vi "Heat1D_Cal Coeff.vi"(9 "a":dbl, 10 "k":dbl=1.0, 11 "Domain":T1) -> (2 "Coefficients":cluster{"r":dbl, "s":dbl, "dt":dbl, "dx":dbl}, 3 "Domain Dup":T1)   [LabVIEW 2017, in "NI_PDE.lvlib"]
uses:
  <vilib>/gmath/NI_PDE.lvlib
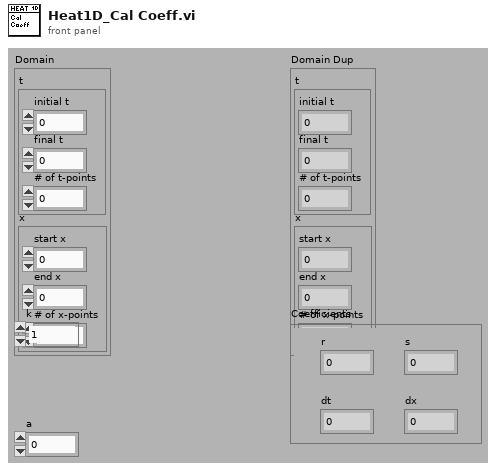
[diagram p1: front panel]
types:
  T1 = cluster{"t":cluster{"initial t":dbl, "final t":dbl, "# of t-points":i32}, "x":cluster{"start x":dbl, "end x":dbl, "# of x-points":i32}}
  T2 = cluster{"initial t":dbl, "final t":dbl, "# of t-points":i32}
  T3 = cluster{"start x":dbl, "end x":dbl, "# of x-points":i32}
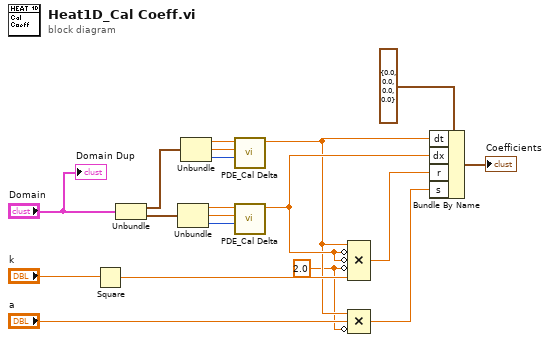
[diagram p0: block diagram]
diagram:
  w3 = 2.0 ("value")
  n1 = Square(x="k") -> (x^2=w7:dbl)
  n2 = Unbundle("Domain") -> ("t"=w19:T2, "x"=w18:T3)
  n3 = Unbundle(w18) -> ("start x"=w14:dbl, "end x"=w12:dbl, "# of x-points"=w13:i32)
  n4 = Unbundle(w19) -> ("initial t"=w17:dbl, "final t"=w16:dbl, "# of t-points"=w15:i32)
  n5 = call <vilib>:"PDE_Cal Delta.vi"("# of points"=w15, "end"=w16, "start"=w17) -> ("delta"=w5:dbl)  [unwired: 8 out]
  n6 = call <vilib>:"PDE_Cal Delta.vi"("# of points"=w13, "end"=w12, "start"=w14) -> ("delta"=w8:dbl)  [unwired: 8 out]
  n7 = Compound Arithmetic op=MULTIPLY(w5, invert w8, invert w8, invert w3, w7) -> (w6:dbl)
  n8 = Compound Arithmetic op=MULTIPLY(w5, "a", invert w3) -> (w2:dbl)
  n9 = Bundle By Name(cluster=cluster{"r":dbl, "s":dbl, "dt":dbl, "dx":dbl} {"r"=0.0, "s"=0.0, "dt"=0.0, "dx"=0.0} ("Coefficients 2"), "dt"=w5, "dx"=w8, "r"=w6, "s"=w2) -> (→"Coefficients":cluster{"r":dbl, "s":dbl, "dt":dbl, "dx":dbl})
  "Domain Dup" <- "Domain"
